vi "GetPanelOrigin.vi"(8 "error in (no error)":errorcluster, 11 "VI in":refnum<vi>) -> (0 "error out":errorcluster, 2 "Origin":T1, 3 "VI out":refnum<vi>)   [LabVIEW 2019, in "ExpandVertical.xctl"]
uses:
  ExpandVertical.xctl
  <vilib>/Utility/miscctls.llb/LVPointTypeDef.ctl
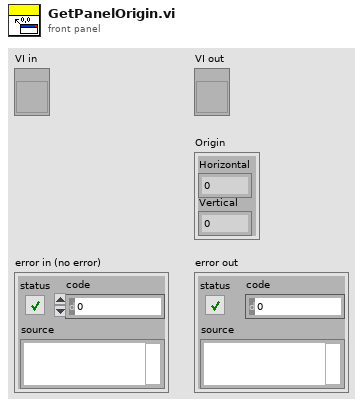
[diagram p1: front panel]
types:
  T1 = typedef "LVPointTypeDef.ctl" = cluster{"Horizontal":i16, "Vertical":i16}
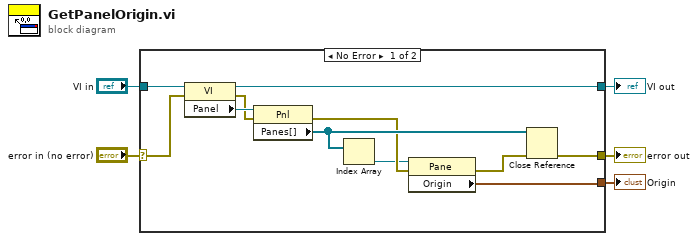
[diagram p0: block diagram]
diagram:
  n1 = case shown="No Error" "error in (no error)" {
    selector: "error in (no error)" -> [w13 w18]
    tunnel: [w16 w17] -> w5
    tunnel: [w15 w18] -> w4
    tunnel: "VI in" -> [w12 w17]
    tunnel: [w6 _] -> w1
    frame No Error {
      n2 = property class="VI"(reference=w12, error in=w13) -> (reference out=w16:refnum<vi>, error out=w8:errorcluster, "Panel"=w9:refnum<vi>)
      n3 = property class="Pnl"(reference=w9, error in=w8) -> (error out=w10:errorcluster, "Panes[]"=w14:refnum<vi>[])  [unwired: 1 out]
      n4 = Index Array(array=w14) -> (element=w7:refnum<vi>)  [unwired: 1 in]
      n5 = property class="Pane"(reference=w7, error in=w10) -> (error out=w11:errorcluster, "Origin"=w6:T1)  [unwired: 1 out]
      n6 = Close Reference(reference=w14, error in (no error)=w11) -> (error out=w15:errorcluster)
    }
    frame Error {
    }
  }
  "VI out" <- w5
  "error out" <- w4
  "Origin" <- w1
